vi "Remove all Cached Files from System.vi"(8 "error in":errorcluster) -> (0 "error out":errorcluster, 1 "Success?":bool)   [LabVIEW 2020, in "ClassLoader.lvlib"]
doc: "Delete all cached config files. \nUse this to remove all traces of ClassLoader usage from application data."
uses:
  ClassLoader.lvlib
  Sub/Ctl/Ctl_Un-load Scope.ctl
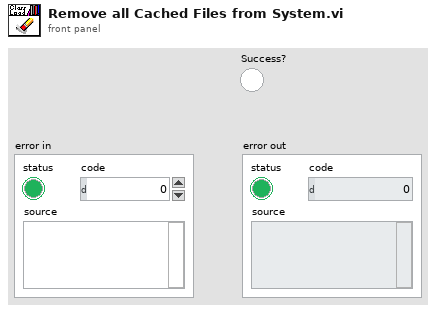
[diagram p1: front panel]
types:
  T1 = typedef "ClassLoader.lvlib/Ctl_Un-load Scope.ctl" = enum16{"Not Paths", "Not Paths nor Hierarchies", "All"}
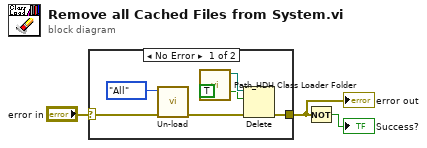
[diagram p0: block diagram]
diagram:
  n1 = case shown="No Error" "error in" {
    selector: "error in" -> [w6 w10]
    tunnel: [w7 w10] -> w2
    frame No Error {
      n2 = call "Un-load.vi"("error in (no error)"=w6, "Scope(Not Paths)"=Ctl_Un-load_Scope."All") -> ("error out"=w5:errorcluster)  [unwired: 9 in]
      n3 = call "Path_HDH Class Loader Folder.vi"() -> ("HDH\\Class Loader path"=w9:path)  [unwired: 11 in]
      n4 = Delete(path (use dialog)=w9, entire hierarchy (F)=TRUE, error in=w5) -> (error out=w7:errorcluster)  [unwired: 2 in, 2 out]
    }
    frame Error {
    }
  }
  "error out" <- w2
  n5 = Not(x=w2) -> (.not. x?=→"Success?":bool)
